vi "Get Node Path Children.vi"(8 "error in (no error)":errorcluster, 10 "Node Path":string, 11 "SDF Ref":refnum<k24>) -> (0 "error out":errorcluster, 2 "Children":string[](array[string]))   [LabVIEW 2016, in "System Mapping Tool.lvlib"]
uses:
  System Mapping Tool.lvlib
  NationalInstruments.VeriStand.SystemDefinitionAPI
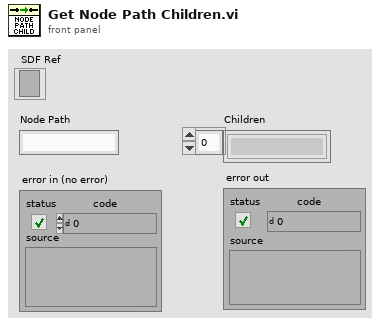
[diagram p1: front panel]
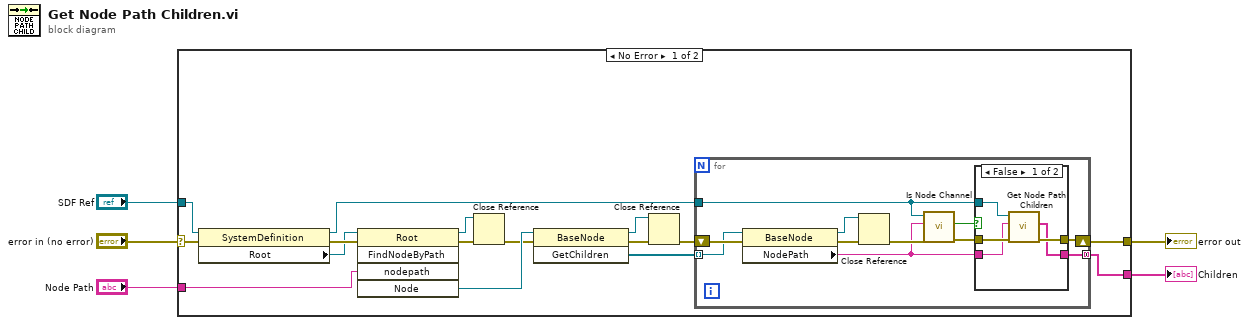
[diagram p0: block diagram]
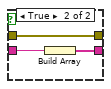
[diagram p2: hidden frame]
diagram:
  n1 = case shown="No Error" "error in (no error)" {
    selector: "error in (no error)" -> [w21 w41]
    tunnel: [w11 w41] -> w4
    tunnel: "SDF Ref" -> [w9 _]
    tunnel: "Node Path" -> [w18 _]
    tunnel: [w10 _] -> w1
    frame No Error {
      n2 = property class="SystemDefinition"(reference=w9, error in=w21) -> (reference out=w8:refnum<k24>, error out=w20:errorcluster, "Root"=w19:refnum<k24>)
      n3 = invoke class="Root" method="FindNodeByPath"(reference=w19, error in=w20, "nodepath"=w18) -> (reference out=w14:refnum<k24>, error out=w16:errorcluster, "Node"=w17:refnum<k24>)  [unwired: 2 in, 2 out]
      n4 = Close Reference(reference=w14, error in (no error)=w16) -> (error out=w15:errorcluster)
      n5 = invoke class="BaseNode" method="GetChildren"(reference=w17, error in=w15) -> (reference out=w6:refnum<k24>, error out=w13:errorcluster, "GetChildren"=w12:refnum<k24>[])  [unwired: 1 in]
      n6 = Close Reference(reference=w6, error in (no error)=w13) -> (error out=w7:errorcluster)
      n7 = for {
        shift-right: [w23] -> w11
        shift-left: w7 -> [w32]
        tunnel: w12 -> [w31] mode=indexing
        tunnel: [w24] -> w10 mode=concatenating
        tunnel: w8 -> [w22]
        n8 = property class="BaseNode"(reference=w31, error in=w32) -> (reference out=w29:refnum<k24>, error out=w30:errorcluster, "NodePath"=w25:string)
        n9 = Close Reference(reference=w29, error in (no error)=w30) -> (error out=w28:errorcluster)
        n10 = call "Is Node Channel.vi"("error in (no error)"=w28, "Node Path"=w25, "SDF Ref"=w22) -> ("error out"=w26:errorcluster, "Is Channel?"=w27:bool)  [unwired: 7 in]
        n11 = case shown="False" w27 {
          tunnel: w26 -> [w37 w38]
          tunnel: w25 -> [w34 w40]
          tunnel: [w35 w39] -> w24
          tunnel: [w36 w38] -> w23
          tunnel: w22 -> [w33 _]
          frame False {
            n12 = call "Get Node Path Children.vi"("error in (no error)"=w37, "Node Path"=w34, "SDF Ref"=w33) -> ("error out"=w36:errorcluster, "Children"=w35:string[])  [unwired: 7 in]
          }
          frame True {
            n13 = Build Array(w40) -> (w39:string[])
          }
        }
      }
    }
    frame Error {
    }
  }
  "error out" <- w4
  "Children" <- w1
